vi "Password.vi"(2 "Admin File Directory":string="C:\\Setup Files\\", 3 "MFC Error":u32) -> ()   [LabVIEW 2014]
panel:
  in  "OK Button":bool
  out "Tab Control":enum32{"System "}(tab)
  in  "Password":string
  in  "Password Input":bool
  # "Admin Menu"
  # "Please Enter Password"
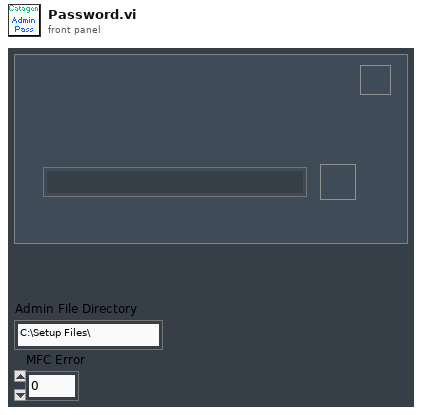
[diagram p1: front panel]
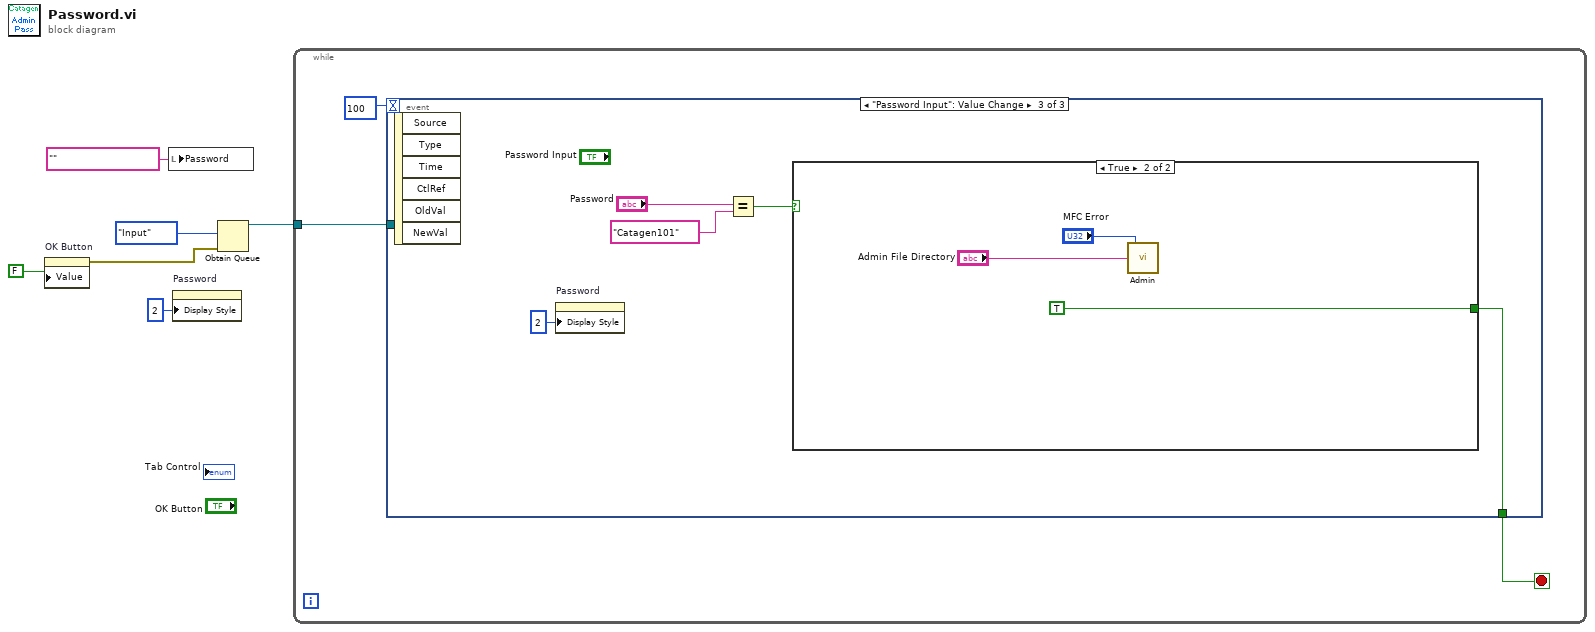
[diagram p0: block diagram]
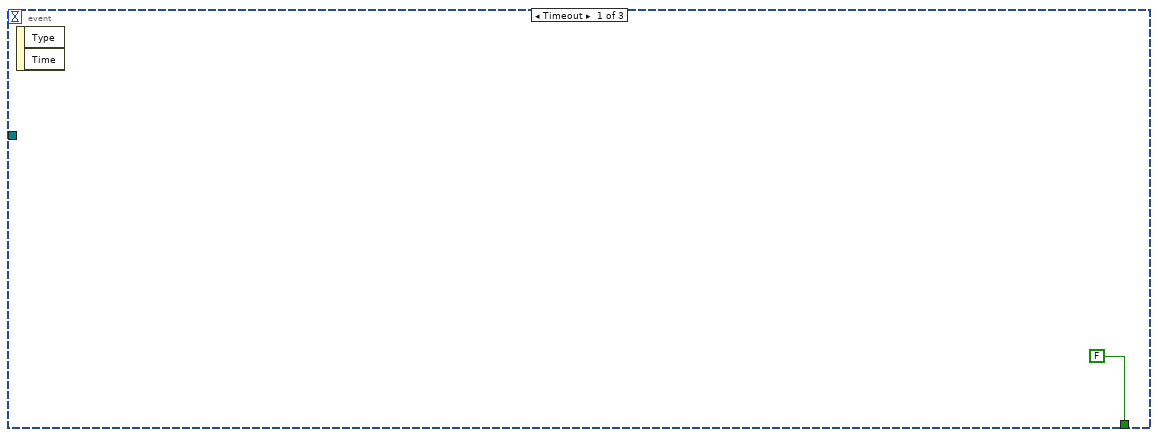
[diagram p2: hidden frame]
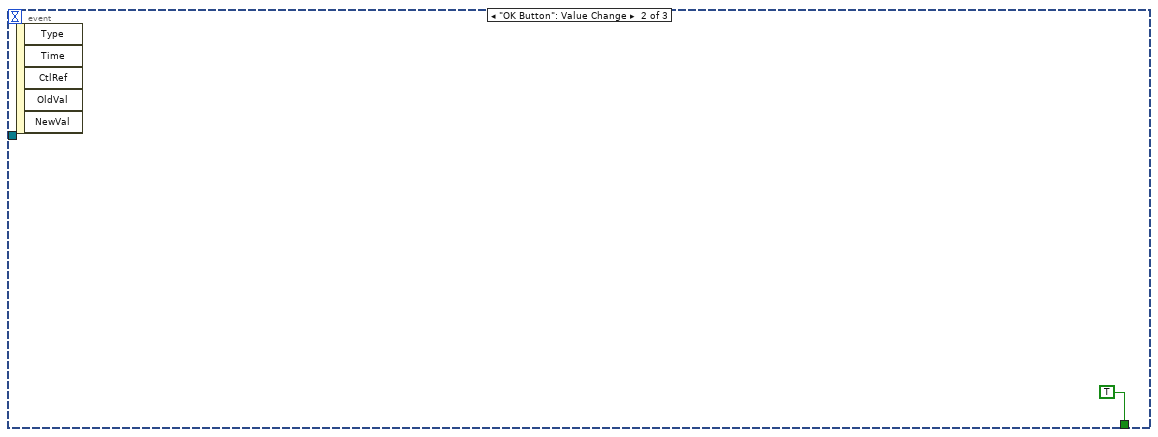
[diagram p3: hidden frame]
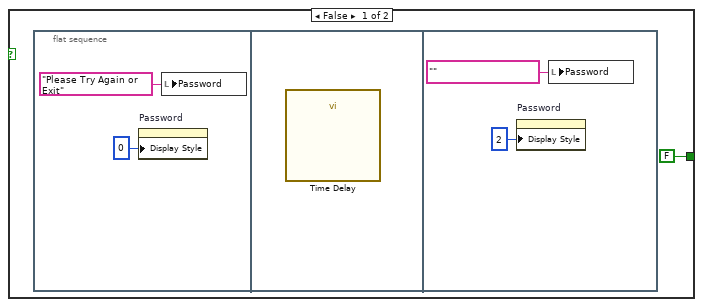
[diagram p4: hidden frame]
diagram:
  n1 = property on="OK Button" class="Bool (strict)"("Value"=FALSE ("OK Button")) -> (error out=w4:errorcluster)  [unwired: 2 in, 1 out]
  n2 = local write "Password"("" ("Password")) -> ()
  n3 = property on="Password" class="Str"("Display Style"=u32 2) -> ()  [unwired: 2 in, 2 out]
  n4 = Obtain Queue(element data type=enum16{"Input", "Check"}."Input", error in (no error)=w4) -> (queue out=w5:refnum<queue>)  [unwired: 3 in, 2 out]
  n5 = while {
    tunnel: w5 -> [w8]
    stop <- w7 stop-if-true
    n6 = event shown="[2] \"Password Input\": Value Change" {
      selector: _ -> [_ _ _]
      dyn-events: _ -> [_ _ _]
      timeout: 100 -> [_ _ _]
      tunnel: w8 -> [_ _ _]
      tunnel: [FALSE TRUE w13] -> w7
      event Timeout {
        n7 = event-data() -> ()  [unwired: 1 in, 2 out]
      }
      event "OK Button": Value Change {
        n8 = event-data() -> ()  [unwired: 1 in, 5 out]
      }
      event "Password Input": Value Change {
        n9 = event-data() -> ()  [unwired: 1 in, 6 out]
        n10 = property on="Password" class="Str"("Display Style"=u32 2) -> ()  [unwired: 2 in, 2 out]
        n11 = Equal?(x="Password", y="Catagen101") -> (x = y?=w14:bool)
        n12 = case shown="True" w14 {
          tunnel: [FALSE TRUE] -> w13
          frame False {
            n13 = flat-sequence {
              frame #0 {
                n14 = property on="Password" class="Str"("Display Style"=u32 0) -> ()  [unwired: 2 in, 2 out]
                n15 = local write "Password"("Please Try Again or Exit" ("Password")) -> ()
              }
              frame #1 {
                n16 = call "Time Delay"() -> ()  [unwired: 11 in, 1 out]
              }
              frame #2 {
                n17 = property on="Password" class="Str"("Display Style"=u32 2) -> ()  [unwired: 2 in, 2 out]
                n18 = local write "Password"("" ("Password")) -> ()
              }
            }
          }
          frame True {
            n19 = call "Admin.vi"("Admin File Directory"="Admin File Directory", "MFC Error"="MFC Error") -> ()  [unwired: 2 in]
          }
        }
      }
    }
  }
